vi "Write Laser Controller.vi"(8 "error in (no error)":errorcluster, 10 "Laser API.lvclass":refnum<class "Laser API.lvclass">, 11 "In":refnum<class "Laser View.lvclass">) -> (0 "error out":errorcluster, 3 "Out":refnum<class "Laser View.lvclass">)   [LabVIEW 2022 SP3, in "Laser View.lvclass"]
uses:
  Laser View.lvclass
  Laser View.lvclass/Laser View.ctl
  Laser Controller api/Laser API.lvclass
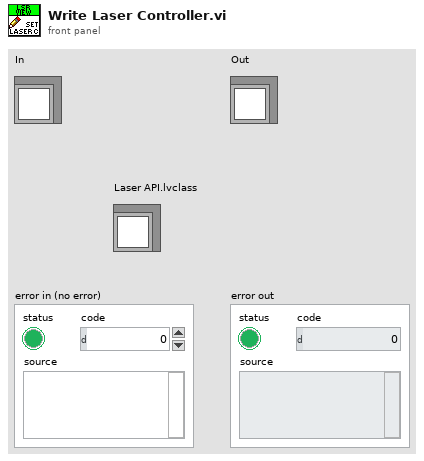
[diagram p1: front panel]
types:
  T1 = typedef "Laser View.lvclass/Data.ctl" = cluster{"Laser API.lvclass":refnum<class "Laser API.lvclass">}
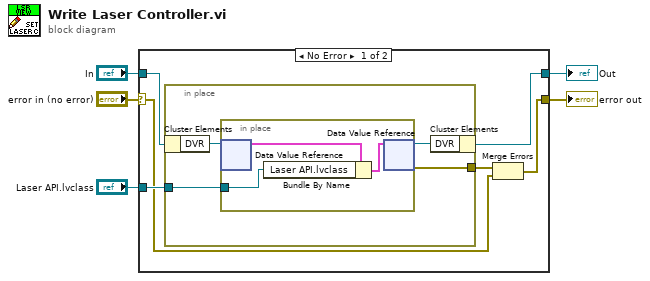
[diagram p0: block diagram]
diagram:
  n1 = case shown="No Error" "error in (no error)" {
    selector: "error in (no error)" -> [w6 w20]
    tunnel: [w7 w20] -> w4
    tunnel: [w11 w19] -> w3
    tunnel: "In" -> [w10 w19]
    tunnel: "Laser API.lvclass" -> [w9 _]
    frame No Error {
      n2 = in-place {
        in-place-border: w9 -> [w13]
        in-place-border: [w12] -> w8
        n3 = in-place-cluster #1(w10) -> ("DVR"=w14:refnum<data-value>)
        n4 = in-place {
          in-place-border: w13 -> [w17]
          n5 = in-place-dvr #2(w14) -> (w16:T1)  [unwired: 1 out]
          n6 = Bundle By Name(cluster=w16, "Laser API.lvclass"=w17) -> (w18:T1)
          n7 = in-place-dvr #2(w18) -> (w15:refnum<data-value>, w12:errorcluster)
        }
        n8 = in-place-cluster #1("DVR"=w15) -> (w11:refnum<class "Laser View.lvclass">)
      }
      n9 = Merge Errors(w8, w6) -> (w7:errorcluster)
    }
    frame Error {
    }
  }
  "Out" <- w3
  "error out" <- w4
